vi "Get Async Status.vi"(8 "error in (no error)":errorcluster, 10 "timeout in ms (0)":i32, 11 "Status in":refnum<queue>) -> (0 "error out":errorcluster, 2 "State":T1, 3 "Status out":refnum<queue>)   [LabVIEW 2011, in "Scan Engine Custom Device.lvlib"]
uses:
  Scan Engine Custom Device.lvlib
  Type Defs/Async State.ctl
  Type Defs/Async Status.ctl
  Globals/Error Strings.vi
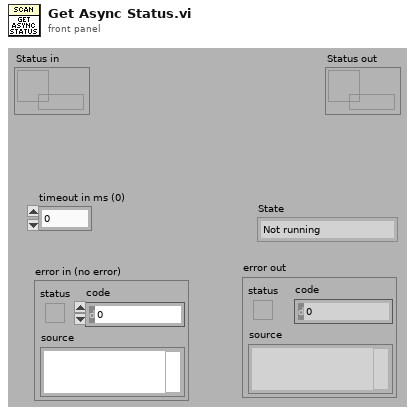
[diagram p1: front panel]
types:
  T1 = typedef "Scan Engine Custom Device.lvlib/Async State.ctl" = enum16{"Not running", "Waiting on start cmd", "Running", "Paused", "Stopped"}
  T2 = typedef "Scan Engine Custom Device.lvlib/Async Status.ctl" = cluster{"State":T1, "error":errorcluster}
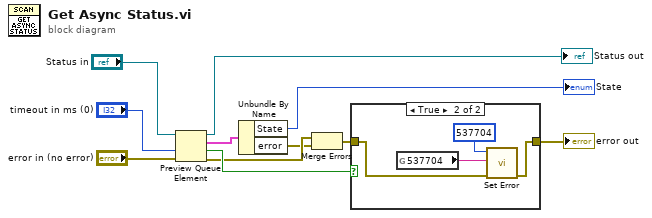
[diagram p0: block diagram]
diagram:
  n1 = Preview Queue Element(queue="Status in", timeout in ms (-1)="timeout in ms (0)", error in (no error)="error in (no error)") -> (queue out=→"Status out":refnum<queue>, element=w11:T2, timed out?=w7:bool, error out=w3:errorcluster)
  n2 = Unbundle By Name(w11) -> ("State"=→"State":T1, "error"=w2:errorcluster)
  n3 = Merge Errors(w3, w2) -> (w1:errorcluster)
  n4 = case shown="True" w7 {
    tunnel: [w12 w16] -> w6
    tunnel: w1 -> [w12 w14]
    frame False {
    }
    frame True {
      n5 = global read "Error Strings.vi" "537704"() -> (w13:string)
      n6 = call "Set Error.vi"("error in (no error)"=w14, "Message"=w13, "Code"=537704 ("code")) -> ("error out"=w16:errorcluster)  [unwired: 8 in]
    }
  }
  "error out" <- w6
